vi "DriveEncoderRevToDist.vi"(6 "Reset_Encoder?":bool, 8 "Invert?":bool, 9 "Wheel_Diameter (In)":dbl, 10 "Counts_Per_Rev":dbl, 11 "Encoder_Rev_Count":dbl) -> (3 "Dist_Travelled (In)":dbl)   [LabVIEW 2016, in "ArgosLib.lvlib"]
uses:
  ArgosLib.lvlib
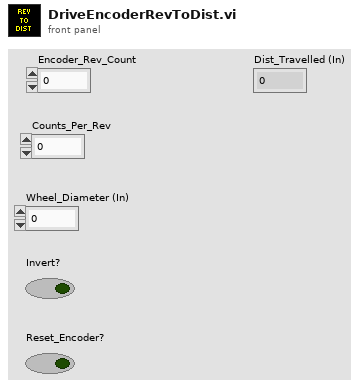
[diagram p1: front panel]
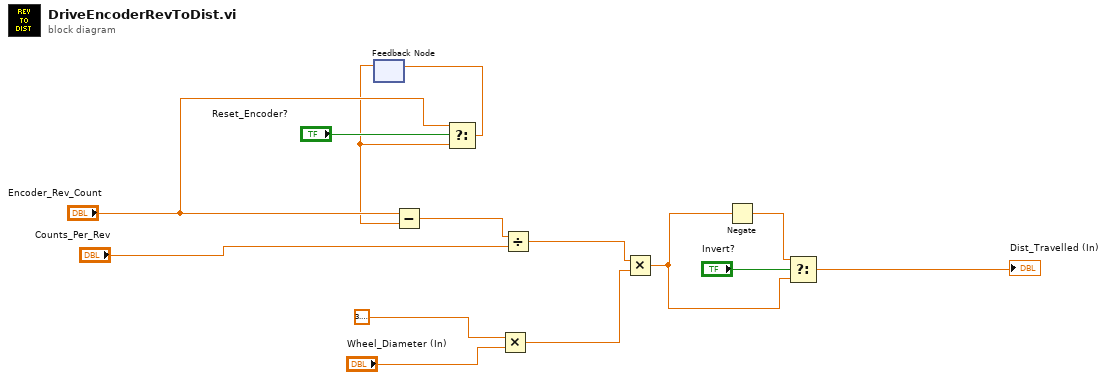
[diagram p0: block diagram]
diagram:
  n1 = feedback #1() -> (w1:dbl)  [unwired: 1 in]
  n2 = Subtract(x="Encoder_Rev_Count", y=w1) -> (x-y=w4:dbl)
  n3 = Select(t="Encoder_Rev_Count", s="Reset_Encoder?", f=w1) -> (s? t:f=w6:dbl)
  n4 = feedback-in #1(w6) -> ()
  n5 = Multiply(x=3.141592653589793, y="Wheel_Diameter (In)") -> (x*y=w12:dbl)
  n6 = Divide(x=w4, y="Counts_Per_Rev") -> (x/y=w2:dbl)
  n7 = Multiply(x=w2, y=w12) -> (x*y=w9:dbl)
  n8 = Negate(x=w9) -> (-x=w10:dbl)
  n9 = Select(t=w10, s="Invert?", f=w9) -> (s? t:f=→"Dist_Travelled (In)":dbl)
